vi "pattern_recognition.vi"(0 "read buffer in":string) -> (2 "read buffer out":string, 3 "Boolean":bool)   [LabVIEW 2016]
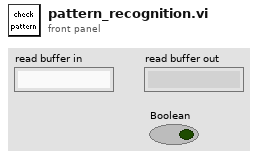
[diagram p1: front panel]
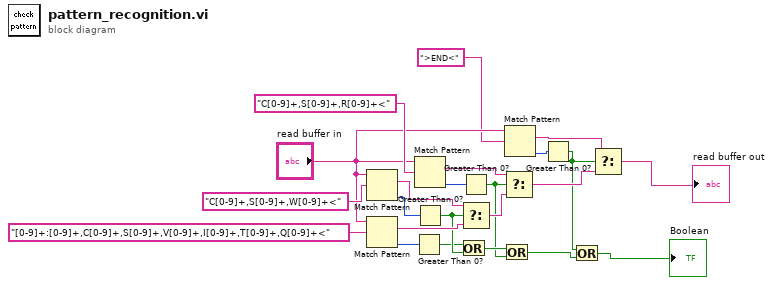
[diagram p0: block diagram]
diagram:
  n1 = Match Pattern(string="read buffer in", regular expression="C[0-9]+,S[0-9]+,W[0-9]+<") -> (match substring=w19:string, offset past match=w15:i32)  [unwired: 1 in, 2 out]
  n2 = Match Pattern(string="read buffer in", regular expression="[0-9]+:[0-9]+,C[0-9]+,S[0-9]+,V[0-9]+,I[0-9]+,T[0-9]+,Q[0-9]+<") -> (match substring=w18:string, offset past match=w11:i32)  [unwired: 1 in, 2 out]
  n3 = Greater Than 0?(x=w11) -> (x > 0?=w10:bool)
  n4 = Match Pattern(string="read buffer in", regular expression="C[0-9]+,S[0-9]+,R[0-9]+<") -> (match substring=w22:string, offset past match=w13:i32)  [unwired: 1 in, 2 out]
  n5 = Greater Than 0?(x=w15) -> (x > 0?=w14:bool)
  n6 = Or(x=w10, y=w14) -> (x .or. y?=w23:bool)
  n7 = Greater Than 0?(x=w13) -> (x > 0?=w12:bool)
  n8 = Select(t=w19, s=w14, f=w18) -> (s? t:f=w21:string)
  n9 = Or(x=w23, y=w12) -> (x .or. y?=w6:bool)
  n10 = Select(t=w22, s=w12, f=w21) -> (s? t:f=w4:string)
  n11 = Match Pattern(string="read buffer in", regular expression=">END<") -> (match substring=w3:string, offset past match=w7:i32)  [unwired: 1 in, 2 out]
  n12 = Greater Than 0?(x=w7) -> (x > 0?=w2:bool)
  n13 = Or(x=w2, y=w6) -> (x .or. y?=→"Boolean":bool)
  n14 = Select(t=w3, s=w2, f=w4) -> (s? t:f=→"read buffer out":string)
